vi "HVBuncher.constructor.vi"(0 "name":string, 2 "data in":string, 5 "error in (no error)":errorcluster) -> (14 "i ref out":refnum<vi>, 16 "data out":string, 19 "error out":errorcluster)   [LabVIEW 2014, in "HVBuncher.lvlib"]
doc: "This is the constructor of a class.\n\nLicense Agreement for this software:\n\nCopyright (C)\nGesellschaft für Schwerionenforschung, GSI\nPlanckstr. 1\n64291 Darmstadt\nGermany\n\nContact: D.Beck@gsi.de \n\nThis program is free software; you can redistribute it and/or modify it under the terms of the \nGNU General Public License as published by the Free Software Foundation; either version 2 of \nthe license, or (at your option) any later version.\n\nThis program is distributed in the hope that it will be useful, but WITHOUT ANY WARRANTY; \nwithout even the implied warranty of MERCHANTABILITY or FITNESS FOR A PARTICULAR PURPOSE. See the GNU General License for more details (http://www.gnu.org).\n\nGesellschaft für Schwerionenforschung, GSI\nPlanckstr. 1, 64291 Darmstadt, Germany\nFor all questions and ideas contact: M.Richter@gsi.de, H.Brand@gsi.de or D.Beck@gsi.de.\nLast update: 16-JUN-2004"
uses:
  HVBuncher.lvlib
  CS_Core/CSApplicationBaseClasses/DeviceBase/DeviceBase.myEventNames.ctl
  CS_Core/CSApplicationBaseClasses/PSChannelBase/PSChannelBase.myEventNames.ctl
  CS_Core/CSSystem/CSSystemLib/CSSystemLib.lvlib
  CS_Core/CSApplicationBaseClasses/PSChannelBase/PSChannelBase.lvlib
  CS_Core/CSApplicationBaseClasses/DeviceBase/DeviceBase.lvlib
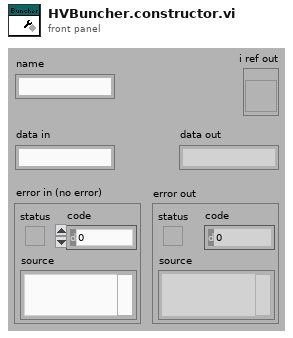
[diagram p1: front panel]
types:
  T1 = enum16{"SetAttribute", "GetAttribute", "CreateAttribute", "DestroyAttribute", "DestroyAllAtributes"}
  T2 = typedef "PSChannelBase.lvlib/PSChannelBase.myEventNames.ctl" = enum16{"lvmsg://EmergencyOff", "lvmsg://SetOnOff", "lvmsg://GetOnOff", "lvmsg://SetVoltage", "lvmsg://GetVoltage", "lvmsg://SetCurrent", "lvmsg://GetCurrent", "lvmsg://SetTripCurrent", "lvmsg://GetTripCurrent", "lvmsg://SetRampUpSpeed", "lvmsg://GetRampUpSpeed", "lvmsg://SetRampDownSpeed", "lvmsg://GetRampDownSpeed", "lvmsg://SetChannelOnOff", "lvmsg://GetChannelOnOff", "lvmsg://SetChannelVoltage", "lvmsg://GetChannelVoltage", "lvmsg://SetChannelCurrent", "lvmsg://GetChannelCurrent", "lvmsg://SetChannelTripCurrent", "lvmsg://GetChannelTripCurrent", "lvmsg://SetChannelRampUpSpeed", "lvmsg://GetChannelRampUpSpeed", "lvmsg://SetChannelRampDownSpeed", "lvmsg://GetChannelRampDownSpeed"}
  T3 = typedef "DeviceBase.lvlib/DeviceBase.myEventNames.ctl" = enum16{"lvmsg://Initialize", "lvmsg://Close", "lvmsg://Configure", "lvmsg://Reset", "lvmsg://IDQuery"}
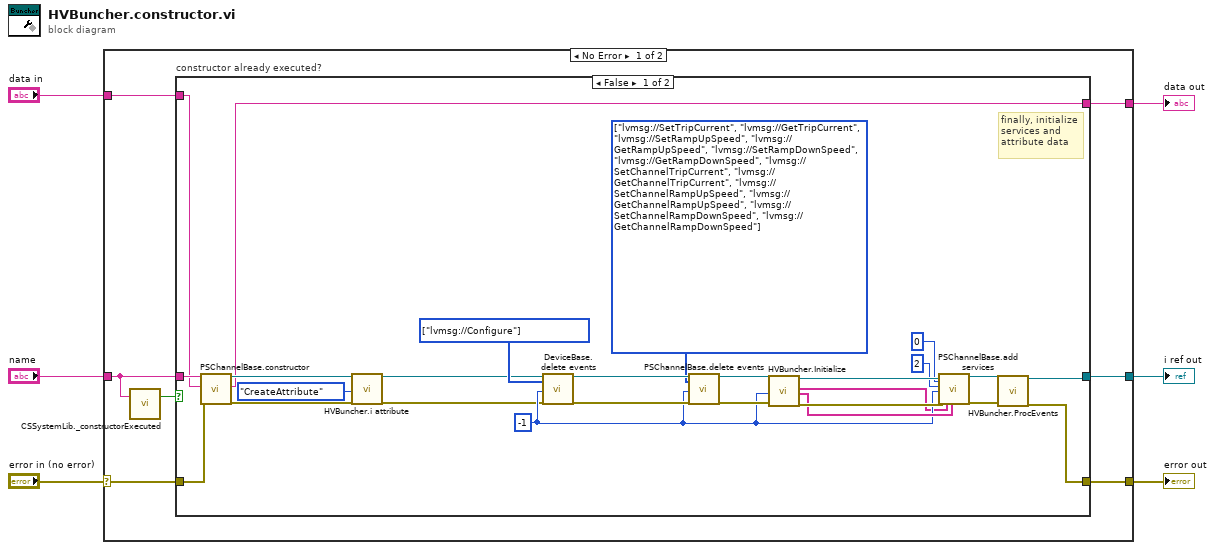
[diagram p0: block diagram]
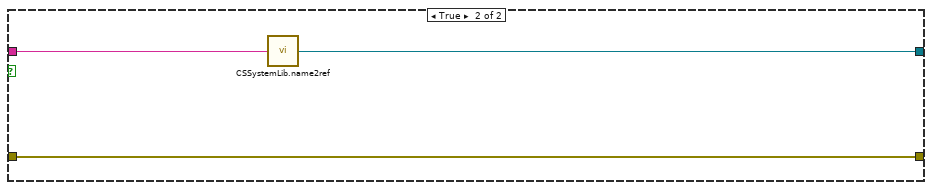
[diagram p2: hidden frame]
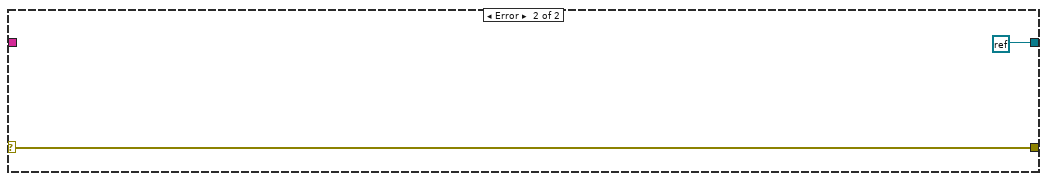
[diagram p3: hidden frame]
diagram:
  n1 = case shown="No Error" "error in (no error)" {
    selector: "error in (no error)" -> [w11 w43]
    tunnel: "name" -> [w10 _]
    tunnel: [w13 refnum<k0> refnum ("Not a Refnum Constant")] -> w5
    tunnel: [w12 w43] -> w4
    tunnel: "data in" -> [w8 _]
    tunnel: [w7 _] -> w1
    frame No Error {
      n2 = call "CSSystemLib._constructorExecuted.vi"("name"=w10) -> ("constructor executed?"=w9:bool)  [unwired: 18 in]
      n3 = case "constructor already executed?" shown="False" w9 {
        tunnel: w10 -> [w36 w42]
        tunnel: [w17 w41] -> w13
        tunnel: [w16 w40] -> w12
        tunnel: w11 -> [w35 w40]
        tunnel: w8 -> [w34 _]
        tunnel: [w29 _] -> w7
        frame False {
          w30 = T2[] [enum."lvmsg://SetTripCurrent", enum."lvmsg://GetTripCurrent", enum."lvmsg://SetRampUpSpeed", enum."lvmsg://GetRampUpSpeed", enum."lvmsg://SetRampDownSpeed", enum."lvmsg://GetRampDownSpeed", enum."lvmsg://SetChannelTripCurrent", enum."lvmsg://GetChannelTripCurrent", enum."lvmsg://SetChannelRampUpSpeed", enum."lvmsg://GetChannelRampUpSpeed", enum."lvmsg://SetChannelRampDownSpeed", enum."lvmsg://GetChannelRampDownSpeed"] items=["lvmsg://EmergencyOff", "lvmsg://SetOnOff", "lvmsg://GetOnOff", "lvmsg://SetVoltage", "lvmsg://GetVoltage", "lvmsg://SetCurrent", "lvmsg://GetCurrent", "lvmsg://SetTripCurrent", "lvmsg://GetTripCurrent", "lvmsg://SetRampUpSpeed", "lvmsg://GetRampUpSpeed", "lvmsg://SetRampDownSpeed", "lvmsg://GetRampDownSpeed", "lvmsg://SetChannelOnOff", "lvmsg://GetChannelOnOff", "lvmsg://SetChannelVoltage", "lvmsg://GetChannelVoltage", "lvmsg://SetChannelCurrent", "lvmsg://GetChannelCurrent", "lvmsg://SetChannelTripCurrent", "lvmsg://GetChannelTripCurrent", "lvmsg://SetChannelRampUpSpeed", "lvmsg://GetChannelRampUpSpeed", "lvmsg://SetChannelRampDownSpeed", "lvmsg://GetChannelRampDownSpeed"] ("events")
          w33 = T3[] [enum."lvmsg://Configure"] items=["lvmsg://Initialize", "lvmsg://Close", "lvmsg://Configure", "lvmsg://Reset", "lvmsg://IDQuery"] ("events")
          w21 = -1 ("ms timeout (10000)")
          # "finally, initialize\nservices and\nattribute data"
          n4 = call "PSChannelBase.constructor.vi"("name"=w36, "data in"=w34, "error in (no error)"=w35) -> ("i ref out"=w39:refnum<vi>, "data out"=w29:string, "error out"=w38:errorcluster)  [unwired: 14 in]
          n5 = call "HVBuncher.i attribute.vi"("VI Refnum"=w39, "Action"=T1."CreateAttribute", "error in (no error)"=w38) -> ("VI Refnum out"=w19:refnum<vi>, "error out"=w18:errorcluster)  [unwired: 14 in, 1 out]
          n6 = call "DeviceBase.delete events.vi"("i ref in"=w19, "events"=w33, "ms timeout (10000)"=w21, "error in (no error)"=w18) -> ("i ref out"=w32:refnum<vi>, "error out"=w31:errorcluster)  [unwired: 13 in, 1 out]
          n7 = call "PSChannelBase.delete events.vi"("i ref in"=w32, "events"=w30, "ms timeout (10000)"=w21, "error in (no error)"=w31) -> ("i ref out"=w28:refnum<vi>, "error out"=w25:errorcluster)  [unwired: 13 in, 1 out]
          n8 = call "HVBuncher.Initialize.vi"("i ref in"=w28, "ms timeout (10000)"=w21, "error in (no error)"=w25) -> ("i ref out"=w27:refnum<vi>, "PhysicalNames"=w20:string[], "LogicalNames"=w24:string[], "error out"=w26:errorcluster)  [unwired: 11 in, 2 out]
          n9 = call "PSChannelBase.add services.vi"("i ref in"=w27, "defaultChannelIndex"=0, "nofChannels"=2, "ms timeout (10000)"=w21, "error in (no error)"=w26, "physicalNames"=w20, "logicalNames"=w24) -> ("i ref out"=w15:refnum<vi>, "error out"=w14:errorcluster)  [unwired: 10 in, 1 out]
          n10 = call "HVBuncher.ProcEvents.vi"("i ref in"=w15, "error in (no error)"=w14) -> ("i ref out"=w17:refnum<vi>, "error out"=w16:errorcluster)  [unwired: 16 in]
        }
        frame True {
          n11 = call "CSSystemLib.name2ref.vi"("name"=w42) -> ("obj refnum"=w41:refnum<vi>)
        }
      }
    }
    frame Error {
    }
  }
  "i ref out" <- w5
  "error out" <- w4
  "data out" <- w1
